vi "FGV_Manage.vi"(8 "error in (no error)":errorcluster, 11 "To do":T5) -> (0 "error out":errorcluster, 3 "All_Communication OUT":T1 {"ConfigurationDatabase"."InactivityTime" format="%.0f seconds"; "ConfigurationDatabase"."TravelTime" format="%.0f seconds"; "ConfigurationDatabase"."DoorClose" format="%.0f seconds"; "ConfigurationDatabase"."DoorOpen" format="%.0f seconds"})   [LabVIEW 2020]
doc: "FGV Manage VI is used to manage configurations as all ref communication for QMH and EVENT and also used for Read/Writte Database Configuration"
uses:
  controls/FGV_To_Do.ctl
  controls/All_Communication_Data.ctl
  controls/Configuration_Database.ctl
  Message Queue/All Message Queues.ctl
  Message Queue/Message Cluster.ctl
  controls/Event_User.ctl
  DataBase/Controls/DB_To_do.ctl
  controls/Share_Data.ctl
  User Event - Stop/User Event - Stop.lvlib
  Message Queue/Message Queue.lvlib
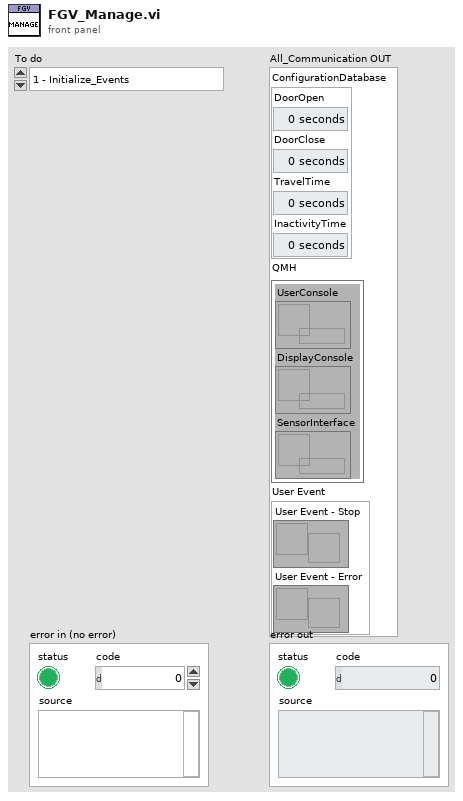
[diagram p1: front panel]
types:
  T1 = typedef "All_Communication_Data.ctl" = cluster{"ConfigurationDatabase":T2, "QMH":T3, "User Event":T4}
  T2 = typedef "Configuration_Database.ctl" = cluster{"DoorOpen":u8, "DoorClose":u8, "TravelTime":u8, "InactivityTime":u8}
  T3 = typedef "Message Queue.lvlib/All Message Queues.ctl" = cluster{"UserConsole":refnum<queue>, "DisplayConsole":refnum<queue>, "SensorInterface":refnum<queue>}
  T4 = typedef "Event_User.ctl" = cluster{"User Event - Stop":refnum<user-event>, "User Event - Error":refnum<user-event>}
  T5 = typedef "FGV_To_Do.ctl" = enum16{"1 - Initialize_Events", "2 - Read_Database", "3 - Initialize QMH", "Save_Database", "Read", "4 - Close_Events", "5 - Close_QMH"}
  T6 = typedef "DB_To_do.ctl" = enum16{"Writte", "Read"}
  T7 = typedef "Share_Data.ctl" = cluster{"ConfigurationDatabase":T2, "User Event":T4}
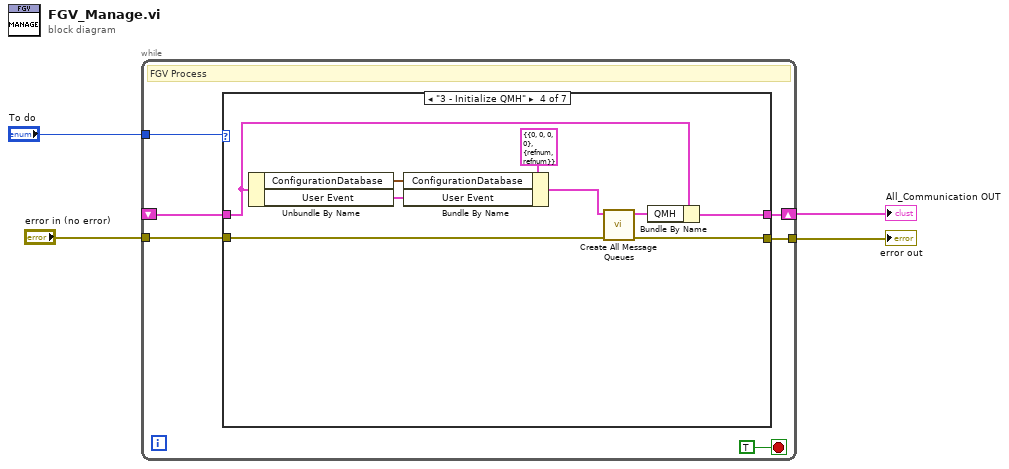
[diagram p0: block diagram]
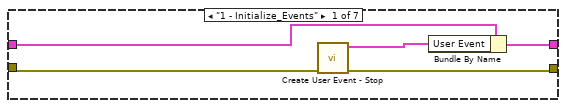
[diagram p2: hidden frame]
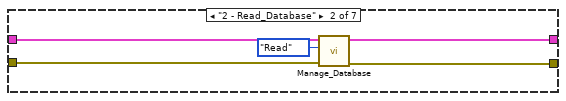
[diagram p3: hidden frame]
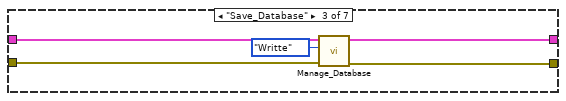
[diagram p4: hidden frame]
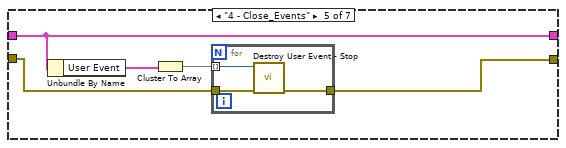
[diagram p5: hidden frame]
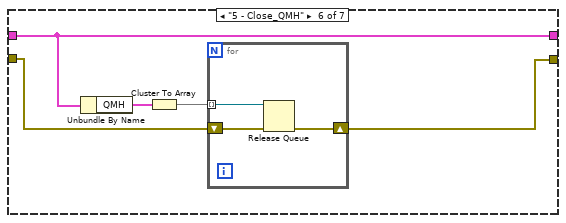
[diagram p6: hidden frame]
diagram:
  n1 = while {
    shift-right: [w9] -> w3
    shift-left: _ -> [w8]
    tunnel: "error in (no error)" -> [w7]
    tunnel: [w6] -> w2
    tunnel: "To do" -> [w5]
    stop <- TRUE stop-if-true
    # "FGV Process"
    n2 = case shown="\"3 - Initialize QMH\"" w5 {
      tunnel: [w12 w19 w24 w32 w37 w45 w52] -> w9
      tunnel: w8 -> [w13 w20 w25 w29 w37 w45 w52]
      tunnel: w7 -> [w15 w18 w23 w34 w39 w47 w51]
      tunnel: [w14 w17 w22 w33 w38 w46 w51] -> w6
      frame "1 - Initialize_Events" {
        n3 = call "Create User Event - Stop.vi"("error in (no error)"=w15) -> ("error out"=w14:errorcluster, "User Event"=w11:T4)  [unwired: 9 in]
        n4 = Bundle By Name(cluster=w13, "User Event"=w11) -> (w12:T1)
      }
      frame "2 - Read_Database" {
        n5 = call "Manage_Database.vi"("error in"=w18, "To_Do"=DB_To_do."Read", "All_Communication IN"=w20) -> ("error out"=w17:errorcluster, "All_Communication OUT"=w19:T1)  [unwired: 7 in]
      }
      frame "Save_Database" {
        n6 = call "Manage_Database.vi"("error in"=w23, "To_Do"=DB_To_do."Writte", "All_Communication IN"=w25) -> ("error out"=w22:errorcluster, "All_Communication OUT"=w24:T1)  [unwired: 7 in]
      }
      frame "3 - Initialize QMH" {
        n7 = Unbundle By Name(w29) -> ("ConfigurationDatabase"=w27:T2, "User Event"=w28:T4)
        n8 = Bundle By Name(cluster=T7 {"ConfigurationDatabase"={"DoorOpen"=0, "DoorClose"=0, "TravelTime"=0, "InactivityTime"=0}, "User Event"={"User Event - Stop"=refnum, "User Event - Error"=refnum}} ("Share_Data"), "ConfigurationDatabase"=w27, "User Event"=w28) -> (w26:T7)
        n9 = call "Create All Message Queues.vi"("error in (no error)"=w34, "Share_Data"=w26) -> ("error out"=w33:errorcluster, "Message Queues out"=w31:T3)  [unwired: 8 in]
        n10 = Bundle By Name(cluster=w29, "QMH"=w31) -> (w32:T1)
      }
      frame "4 - Close_Events" {
        n11 = Unbundle By Name(w37) -> ("User Event"=w36:T4)
        n12 = Cluster To Array(cluster=w36) -> (array=w35:refnum<user-event>[])
        n13 = for {
          tunnel: w39 -> [w42]
          tunnel: [w41] -> w38
          tunnel: w35 -> [w40] mode=indexing
          n14 = call "Destroy User Event - Stop.vi"("error in (no error)"=w42, "User Event - Stop"=w40) -> ("error out"=w41:errorcluster)  [unwired: 9 in]
        }
      }
      frame "5 - Close_QMH" {
        n15 = Unbundle By Name(w45) -> ("QMH"=w44:T3)
        n16 = Cluster To Array(cluster=w44) -> (array=w43:refnum<queue>[])
        n17 = for {
          shift-right: [w49] -> w46
          shift-left: w47 -> [w50]
          tunnel: w43 -> [w48] mode=indexing
          n18 = Release Queue(queue=w48, error in (no error)=w50) -> (error out=w49:errorcluster)  [unwired: 1 in, 2 out]
        }
      }
      frame "Read", Default {
      }
    }
  }
  "All_Communication OUT" <- w3
  "error out" <- w2
